vi "Register gRPC Methods.vi"(8 "error in (no error)":errorcluster, 11 "gRPC service in":refnum<class "Template.lvclass">) -> (0 "error out":errorcluster, 3 "gRPC service out":refnum<class "Template.lvclass">)   [LabVIEW 2021, in "Template_server.lvlib" / "Template.lvclass"]
uses:
  Template.lvclass
  typeDefs/Server Internal UEs.ctl
  typeDefs/Server Internal Message.ctl
  typeDefs/Server gRPC UEs.ctl
  <vilib>/gRPC/LabVIEW gRPC Library/Server API/typeDefs/gRPCId Cluster.ctl
  <vilib>/gRPC/LabVIEW gRPC Library/Shared/grpcId.ctl
  Template.lvclass/Template.ctl
  <vilib>/gRPC/LabVIEW gRPC Library/grpc-lvsupport-release.lvlib
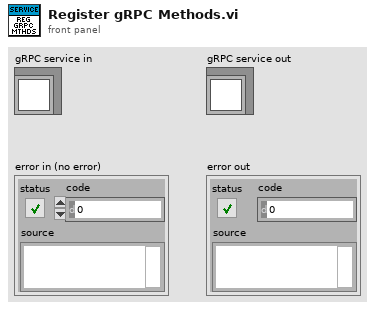
[diagram p1: front panel]
types:
  T1 = typedef "Template_server.lvlib/Template.lvclass/Server gRPC UEs.ctl" = cluster{"Template SetNumeric gRPC UE":refnum<user-event>, "Template GetResult gRPC UE":refnum<user-event>, "Template GetStatistics gRPC UE":refnum<user-event>}
  T2 = typedef "Template_server.lvlib/Template.lvclass/Server Internal UEs.ctl" = cluster{"Template SetNumeric Internal UE":refnum<user-event>, "Template GetResult Internal UE":refnum<user-event>, "Template GetStatistics Internal UE":refnum<user-event>}
  T3 = typedef "grpc-lvsupport-release.lvlib/grpcId.ctl" = u64
  T4 = typedef "Template_server.lvlib/Template.lvclass/Server Internal Message UE.ctl" = refnum<user-event>
  T5 = typedef "grpc-lvsupport-release.lvlib/gRPCId Cluster UE.ctl" = refnum<user-event>
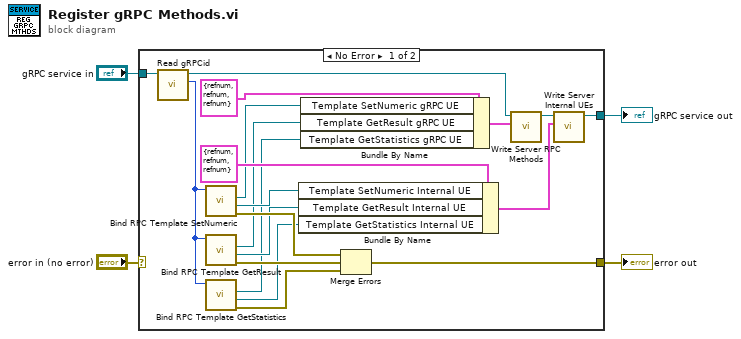
[diagram p0: block diagram]
diagram:
  n1 = case shown="No Error" "error in (no error)" {
    selector: "error in (no error)" -> [_ w24]
    tunnel: "gRPC service in" -> [w15 w25]
    tunnel: [w23 w24] -> w3
    tunnel: [w22 w25] -> w2
    frame No Error {
      n2 = call-dynamic "Read gRPCid.vi"("gRPC service in"=w15) -> ("gRPCid"=w14:T3, "gRPC service out"=w16:refnum<class "Template.lvclass">)  [unwired: 8 in, 1 out]
      n3 = call "Bind RPC Template SetNumeric.vi"("gRPCid server in"=w14) -> ("error out"=w13:errorcluster, "Template SetNumeric Internal UE"=w12:T4, "Template SetNumeric gRPC UE"=w11:T5)  [unwired: 7 in, 1 out]
      n4 = call "Bind RPC Template GetResult.vi"("gRPCid server in"=w14) -> ("error out"=w10:errorcluster, "Template GetResult Internal UE"=w8:T4, "Template GetResult gRPC UE"=w9:T5)  [unwired: 7 in, 1 out]
      n5 = call "Bind RPC Template GetStatistics.vi"("gRPCid server in"=w14) -> ("error out"=w7:errorcluster, "Template GetStatistics Internal UE"=w5:T4, "Template GetStatistics gRPC UE"=w6:T5)  [unwired: 7 in, 1 out]
      n6 = Bundle By Name ("Bundle Internal UEs")(cluster=T2 {"Template SetNumeric Internal UE"=refnum, "Template GetResult Internal UE"=refnum, "Template GetStatistics Internal UE"=refnum} ("Server Internal UEs"), "Template SetNumeric Internal UE"=w12, "Template GetResult Internal UE"=w8, "Template GetStatistics Internal UE"=w5) -> (w21:T2)
      n7 = Bundle By Name ("Bundle gRPC UEs")(cluster=T1 {"Template SetNumeric gRPC UE"=refnum, "Template GetResult gRPC UE"=refnum, "Template GetStatistics gRPC UE"=refnum} ("gRPC Server Method Events"), "Template SetNumeric gRPC UE"=w11, "Template GetResult gRPC UE"=w9, "Template GetStatistics gRPC UE"=w6) -> (w18:T1)
      n8 = Merge Errors(w13, w10, w7) -> (w23:errorcluster)
      n9 = call "Write Server RPC Methods.vi"("Server RPC Methods"=w18, "gRPC service in"=w16) -> ("gRPC service out"=w19:refnum<class "Template.lvclass">)  [unwired: 8 in, 1 out]
      n10 = call "Write Server Internal UEs.vi"("Server Internal UEs"=w21, "gRPC service in"=w19) -> ("gRPC service out"=w22:refnum<class "Template.lvclass">)  [unwired: 8 in, 1 out]
    }
    frame Error {
    }
  }
  "error out" <- w3
  "gRPC service out" <- w2
